vi "ShanTen.vi"(1 "Count":u16[](array[numeric])) -> (0 "ShanTen":i16)   [LabVIEW 2025]
panel:
  out "Target":u16
  out "Pair":u16
  out "Taatsu":u16
  out "Meld":u16
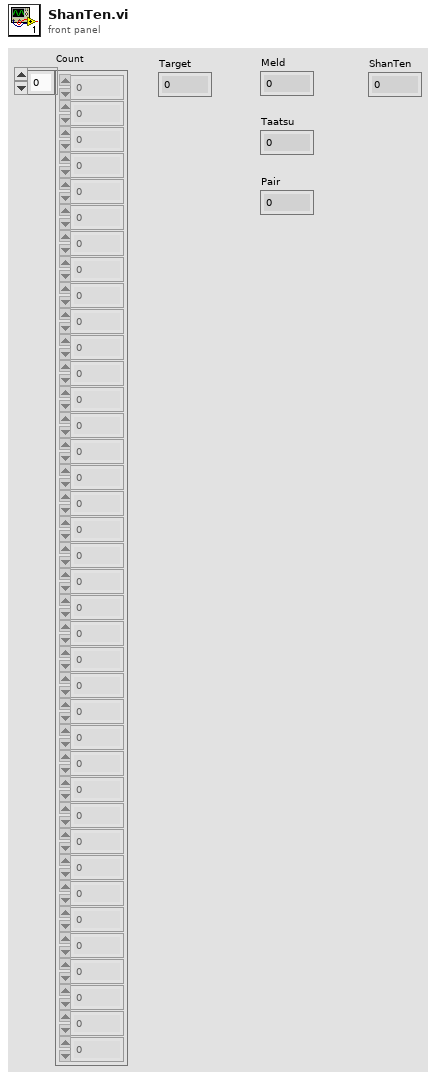
[diagram p1: front panel]
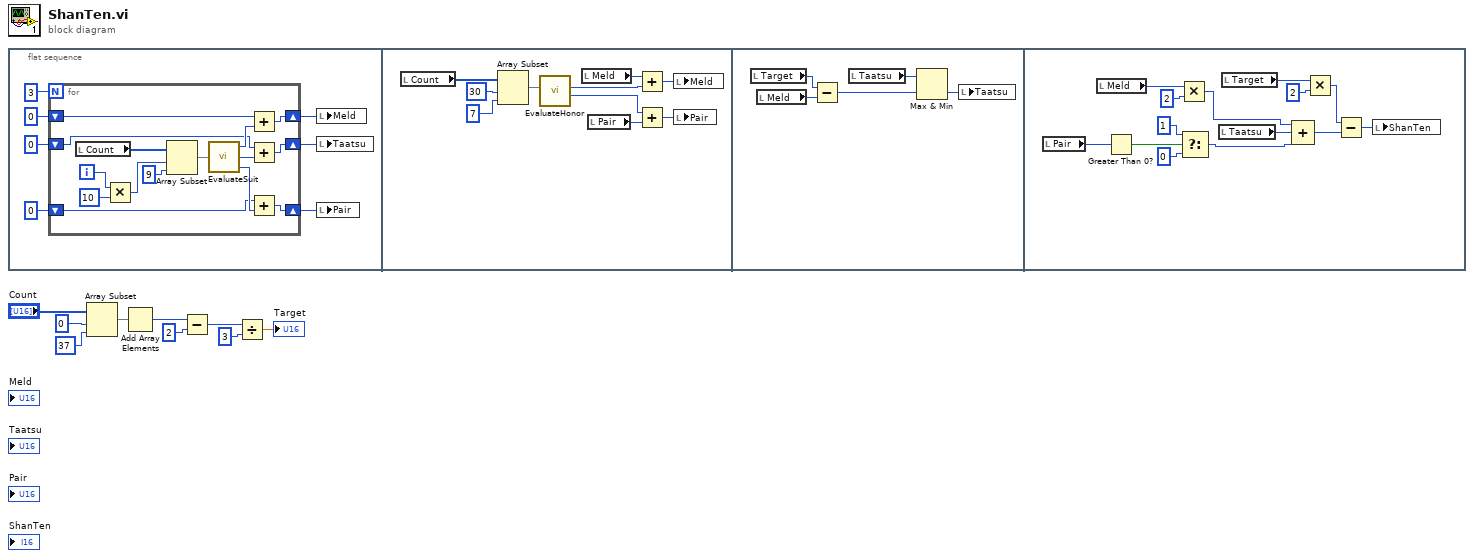
[diagram p0: block diagram]
diagram:
  n1 = flat-sequence {
    frame #0 {
      n2 = for {
        N: 3 -> [_]
        shift-right: [w25] -> w12
        shift-left: u16 0 ("Meld") -> [w21]
        shift-right: [w24] -> w11
        shift-left: u16 0 ("Taatsu") -> [w19]
        shift-right: [w23] -> w10
        shift-left: u16 0 ("Pair") -> [w17]
        i -> [w30]
        n3 = local read "Count"() -> (w26:u16[])
        n4 = Multiply(x=w30, y=10) -> (x*y=w31:i32)
        n5 = Array Subset(array=w26, index=w31, length=9) -> (w27:u16[])
        n6 = call "EvaluateSuit.vi"("Count"=w27) -> ("Pair"=w18:u16, "Taatsu"=w20:u16, "Meld"=w22:u16)  [unwired: 2 in]
        n7 = Add(x=w21, y=w22) -> (x+y=w25:u16)
        n8 = Add(x=w19, y=w20) -> (x+y=w24:u16)
        n9 = Add(x=w17, y=w18) -> (x+y=w23:u16)
      }
      n10 = local write "Meld"(w12) -> ()
      n11 = local write "Taatsu"(w11) -> ()
      n12 = local write "Pair"(w10) -> ()
    }
    frame #1 {
      n13 = local read "Count"() -> (w41:u16[])
      n14 = Array Subset(array=w41, index=30, length=7) -> (w38:u16[])
      n15 = call "EvaluateHonor.vi"("Count"=w38) -> ("Pair"=w37:u16, "Meld"=w32:u16)  [unwired: 9 in]
      n16 = local read "Meld"() -> (w34:u16)
      n17 = local read "Pair"() -> (w36:u16)
      n18 = Add(x=w34, y=w32) -> (x+y=w33:u16)
      n19 = Add(x=w37, y=w36) -> (x+y=w35:u16)
      n20 = local write "Meld"(w33) -> ()
      n21 = local write "Pair"(w35) -> ()
    }
    frame #2 {
      n22 = local read "Target"() -> (w44:u16)
      n23 = local read "Meld"() -> (w43:u16)
      n24 = Subtract(x=w44, y=w43) -> (x-y=w42:u16)
      n25 = local read "Taatsu"() -> (w46:u16)
      n26 = Max & Min(x=w46, y=w42) -> (min(x,y)=w45:u16)  [unwired: 1 out]
      n27 = local write "Taatsu"(w45) -> ()
    }
    frame #3 {
      n28 = local read "Pair"() -> (w50:u16)
      n29 = local read "Meld"() -> (w51:u16)
      n30 = Greater Than 0?(x=w50) -> (x > 0?=w58:bool)
      n31 = Multiply(x=w51, y=u16 2) -> (x*y=w49:u16)
      n32 = Select(t=1, s=w58, f=0) -> (s? t:f=w47:i32)
      n33 = local read "Taatsu"() -> (w48:u16)
      n34 = local read "Target"() -> (w54:u16)
      n35 = Compound Arithmetic op=ADD(w49, w48, w47) -> (w56:i32)
      n36 = Multiply(x=w54, y=u16 2) -> (x*y=w55:u16)
      n37 = Subtract(x=w55, y=w56) -> (x-y=w57:i32)
      n38 = local write "ShanTen"(w57) -> ()
    }
  }
  n39 = Array Subset(array="Count", index=0, length=37) -> (w3:u16[])
  n40 = Add Array Elements(numeric array=w3) -> (sum=w9:u16)
  n41 = Subtract(x=w9, y=2) -> (x-y=w7:i32)
  n42 = Divide(x=w7, y=3) -> (x/y=→"Target":dbl)
